vi "PrepForScan.vi"(0 "Motion Settings In":T1={"No Motion?"=FALSE, "Motion System"=enum."NI 735x", "Motion Bd ID"=1, "Motion Profile"="SMAC1", "# Axis"=1, "Reverse Z axis?"=TRUE, "SMAC Axis"=0, "scan pair"=enum."y-(x) scan", "RT fps"=6.0, "Steps per mm"=[1000, 1000, 1000, 1000], "Motor Parameters"={"velocity ct/s"=[10000.0, 10000.0, 10000.0, 50000.0], "accel ct/s^2"=[50000.0, 50000.0, 50000.0, 200000.0]}, "One Way Scan"=FALSE, "Reverse One Way Scan"=FALSE, "Global Position (mm)"=[], "Plane"=0, "Distance between\nscan lines (um)"=0.0, "Distance between\nscan planes (um)"=0.0, "number of scan planes"=1, "Total steps in line"=0, "Xtra plane\ndistance  (um)"=100, "Xtra planes "=1, "Add Axis"=FALSE, "overshoot cts"=200, "BKPT Shift"=0, "Scan Start Time (ms)"=0, "ESP VISA"="GPIB::1::INSTR", "3rd Axis"=1, "GL Ref Out"=refnum, "Galil Address"=""} {"3rd Axis" items=["x", "y", "z", "w"]; "Xtra planes" min=1; "Xtra plane\ndistance  (um)" min=0; "Distance between\nscan planes (um)" format="%.2f"; "Distance between\nscan lines (um)" format="%.2f"; "SMAC Axis" items=["None"=0, "Axis 1"=1, "Axis 2"=2, "Axis 3"=3, "Axis 4"=4, "Axis 5"=5, "Axis 6"=6, "Axis 7"=7, "Axis 8"=8, "Vector Space 1"=17, "Vector Space 2"=18, "Vector Space 3"=19, "Vector Space 4"=20]; "Motion Bd ID" min=1 max=32 step=1}, 1 "Pause?":bool, 7 "SMAC?":bool, 9 "Scan Axis":i8, 11 "MoveBack?":bool, 12 "Digitizer Settings":T5={"Digitizer delay (us) "=0.0, "rf points per line"=0, "lines per plane"=0, "Samp Rate (Hz)"=0.0, "Additional dig delay (us)"=0.0, "Voltage Scale"=0.0, "Pre-Looks"=0, "Offset delay (us)"=0.0, "bits A/D"=0, "Avg Num"=0, "DigTimeOut"=0.0, "Rel Dig Delay"=0.0, "Dig Ch"=0, "LeCroyCluster"={"LeCroy Channels"=[], "LC read pt offset"=0.0, "Sweep Avg"=FALSE}, "Main Digitizer"=enum."NI Digitizer", "Dig Config"=enum."Single channel", "Digitizer ID Cluster"={"Acqiris/Alazar/SP ID"=[], "NI Instr Handles"=[], "LeCroy VISA"="", "GaGe Handle"={"Handle"=0, "Sample size"=0, "Resolution"=0, "Offset"=0, "Channels"=0, "Boards"=0}, "ATS Ref"="ATS9350", "Acqiris Address"=["PCI::INSTR0"], "ADQRef"=refnum, "adq_cu_ptr"=refnum}, "Trigger Settings"={"Trig Source"=1, "Trig Coupling"=0, "Trig Slope"=0, "Level (mV)"=1500.0}, "Bulk Acq"=FALSE, "Bulk Start Indexes"=[], "Data Ref RF"=refnum, "NI ID/Channel"=[], "Total Dig CH"=1, "Xtra Ann Trig delay (us)"=10.0, "Fix Z Delay?"=FALSE, "One Way Transmission?"=FALSE, "Data Ref Log"=refnum} {"Trigger Settings"."Trig Slope" items=["Positive", "Negative"]; "Trigger Settings"."Level (mV)" format="%.2f"; "Trigger Settings"."Trig Coupling" items=["DC 1 MOhm", "AC 1 MOhm", "DC 50 Ohm", "AC 50 Ohm"]; "Trigger Settings"."Trig Source" items=["Chan 1", "External"]; "Rel Dig Delay" format="%.2f"; "DigTimeOut" format="%.2f"; "Avg Num" min=1; "Offset delay (us)" format="%.2f"; "Additional dig delay (us)" format="%.2f"; "Digitizer delay (us)" format="%.2f"}) -> (4 "Counts":dbl, 6 "Axis Resource out":u16(ring) items=["Axis Control"=0, "Axis 1"=1, "Axis 2"=2, "Axis 3"=3, "Axis 4"=4, "Axis 5"=5, "Axis 6"=6, "Axis 7"=7, "Axis 8"=8, "Vector Space Control"=16, "Vector Space 1"=17, "Vector Space 2"=18, "Vector Space 3"=19, "Vector Space 4"=20, "Encoder Control"=32, "Encoder 1"=33, "Encoder 2"=34, "Encoder 3"=35, "Encoder 4"=36, "Encoder 5"=37, "Encoder 6"=38, "Encoder 7"=39, "Encoder 8"=40, "DAC Channel 1"=49, "DAC Channel 2"=50, "DAC Channel 3"=51, "DAC Channel 4"=52, "DAC Channel 5"=53, "DAC Channel 6"=54, "DAC Channel 7"=55, "DAC Channel 8"=56, "Stepper Output 1"=65, "Stepper Output 2"=66, "Stepper Output 3"=67, "Stepper Output 4"=68, "Stepper Output 5"=69, "Stepper Output 6"=70, "Stepper Output 7"=71, "Stepper Output 8"=72, "ADC Channel 1"=81, "ADC Channel 2"=82, "ADC Channel 3"=83, "ADC Channel 4"=84, "ADC Channel 5"=85, "ADC Channel 6"=86, "ADC Channel 7"=87, "ADC Channel 8"=88], 8 "Bd ID Out":u8, 10 "Program ID":u8 format="%.0x", 14 "Axis Move Info":cluster{"Resource Output":u16, "Position":i32} {"Resource Output" items=["Axis Control"=0, "Axis 1"=1, "Axis 2"=2, "Axis 3"=3, "Axis 4"=4, "Axis 5"=5, "Axis 6"=6, "Axis 7"=7, "Axis 8"=8, "Vector Space Control"=16, "Vector Space 1"=17, "Vector Space 2"=18, "Vector Space 3"=19, "Vector Space 4"=20, "Encoder Control"=32, "Encoder 1"=33, "Encoder 2"=34, "Encoder 3"=35, "Encoder 4"=36, "Encoder 5"=37, "Encoder 6"=38, "Encoder 7"=39, "Encoder 8"=40, "DAC Channel 1"=49, "DAC Channel 2"=50, "DAC Channel 3"=51, "DAC Channel 4"=52, "DAC Channel 5"=53, "DAC Channel 6"=54, "DAC Channel 7"=55, "DAC Channel 8"=56, "Stepper Output 1"=65, "Stepper Output 2"=66, "Stepper Output 3"=67, "Stepper Output 4"=68, "Stepper Output 5"=69, "Stepper Output 6"=70, "Stepper Output 7"=71, "Stepper Output 8"=72, "ADC Channel 1"=81, "ADC Channel 2"=82, "ADC Channel 3"=83, "ADC Channel 4"=84, "ADC Channel 5"=85, "ADC Channel 6"=86, "ADC Channel 7"=87, "ADC Channel 8"=88]}, 15 "error out":errorcluster)   [LabVIEW 2022 SP3]
uses:
  Digitizers/-DigitizerRoutines/DigitizerSettings.ctl
  Digitizers/-DigitizerRoutines/Digitizer.ctl
  Digitizers/-DigitizerRoutines/DigConfig.ctl
  Digitizers/-DigitizerRoutines/DigitizerID.ctl
  C:/Windows/System32/ADQAPI_dotNet_helper.dll
  MotionParameters.ctl
  MotionSys.ctl
  -MotionRoutines/ScanAxis.ctl
  -MotionRoutines/3rdAxis.ctl
  Galil/Command Menu.ctl
  <instrlib>/Newport ESP301/Newport ESP301.lvlib
  <vilib>/Motion/FlexMotion/CustomControls/CustomControls.llb/Program.flx
  <vilib>/Motion/FlexMotion/CustomControls/CustomControls.llb/Axis To Control.flx
panel:
  # "1-D and 2-D B scan settings"
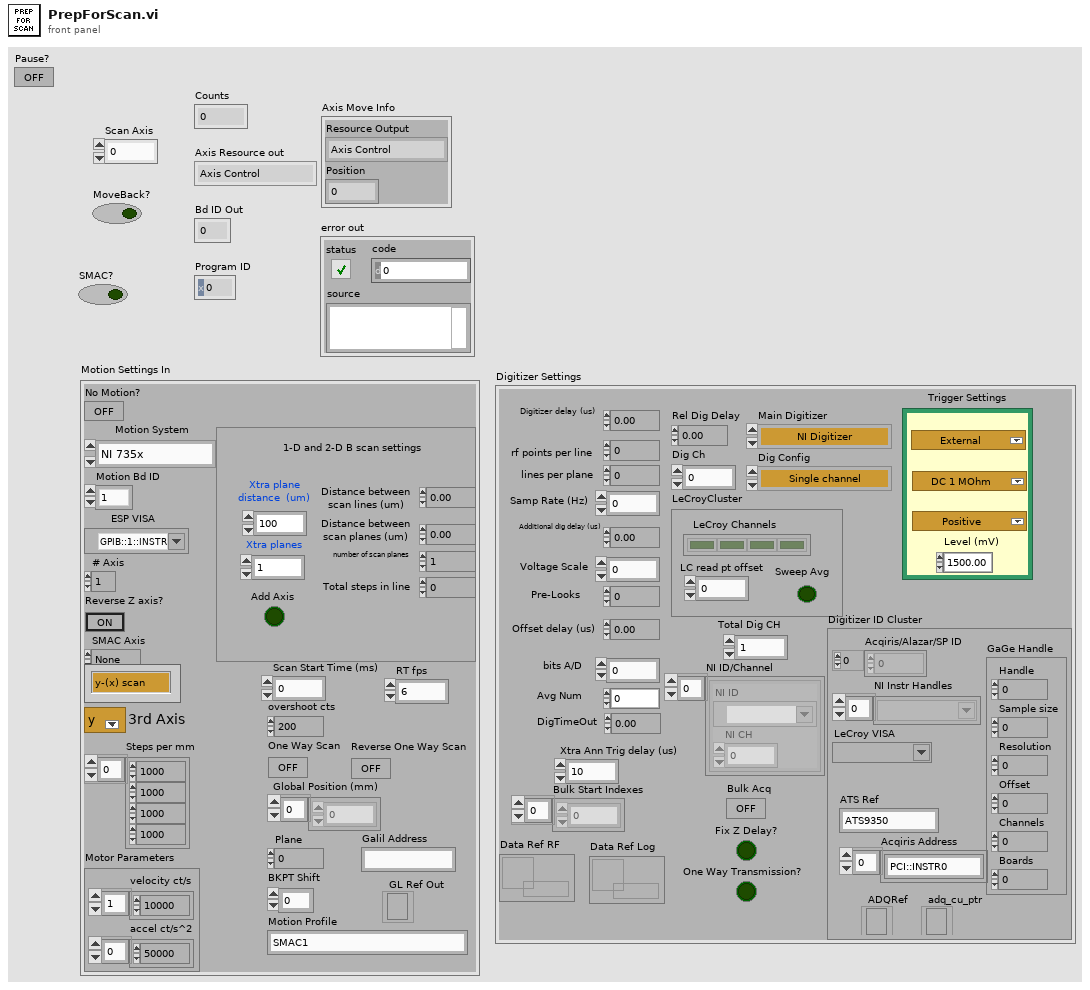
[diagram p1: front panel]
types:
  T1 = typedef "MotionParameters.ctl" = cluster{"No Motion?":bool, "Motion System":T2, "Motion Bd ID":u8, "Motion Profile":string, "# Axis":i8, "Reverse Z axis?":bool, "SMAC Axis":u16, "scan pair":T3, "RT fps":sgl, "Steps per mm":i32[], "Motor Parameters":cluster{"velocity ct/s":dbl[], "accel ct/s^2":dbl[]}, "One Way Scan":bool, "Reverse One Way Scan":bool, "Global Position (mm)":dbl[], "Plane":i32, "Distance between\nscan lines (um)":sgl, "Distance between\nscan planes (um)":sgl, "number of scan planes":i32, "Total steps in line":i32, "Xtra plane\ndistance  (um)":i32, "Xtra planes ":i32, "Add Axis":bool, "overshoot cts":i32, "BKPT Shift":i32, "Scan Start Time (ms)":u32, "ESP VISA":refnum<visa-resource-name>, "3rd Axis":T4, "GL Ref Out":refnum<k7>, "Galil Address":string}
  T2 = typedef "MotionSys.ctl" = enum16{"MM3000", "NI 735x", "Newport ESP", "No Motion Card", "Galil"}
  T3 = typedef "ScanAxis.ctl" = enum16{"y-(x) scan", "x-(y) scan", "z-(x) scan", "z-(y) scan", "y-(z) scan", "x-(z) scan", "w-(x) scan", "w-(y) scan", "w-(z) scan", "x-(w) scan", "y-(w) scan", "z-(w) scan"}
  T4 = typedef "3rdAxis.ctl" = u16
  T5 = typedef "DigitizerSettings.ctl" = cluster{"Digitizer delay (us) ":dbl, "rf points per line":i32, "lines per plane":i32, "Samp Rate (Hz)":dbl, "Additional dig delay (us)":dbl, "Voltage Scale":dbl, "Pre-Looks":i32, "Offset delay (us)":dbl, "bits A/D":i8, "Avg Num":i32, "DigTimeOut":sgl, "Rel Dig Delay":sgl, "Dig Ch":i32, "LeCroyCluster":cluster{"LeCroy Channels":bool[], "LC read pt offset":dbl, "Sweep Avg":bool}, "Main Digitizer":T6, "Dig Config":T7, "Digitizer ID Cluster":T8, "Trigger Settings":cluster{"Trig Source":u16, "Trig Coupling":u16, "Trig Slope":u16, "Level (mV)":dbl}, "Bulk Acq":bool, "Bulk Start Indexes":i32[], "Data Ref RF":refnum<data-value>, "NI ID/Channel":cluster{"NI ID":refnum<k15>, "NI CH":i32}[], "Total Dig CH":i32, "Xtra Ann Trig delay (us)":dbl, "Fix Z Delay?":bool, "One Way Transmission?":bool, "Data Ref Log":refnum<data-value>}
  T6 = typedef "Digitizer.ctl" = enum16{"Acqiris Digitizer", "NI Digitizer", "LeCroy", "GaGe", "AlazarTech", "No Digitizer", "Teledyne"}
  T7 = typedef "DigConfig.ctl" = enum16{"Single channel", "2 Chans w/ 2 Acqiris", "2 Chans w/ 1 Acqiris", "5-CH Pulser New", "5-CH pulser w/ ann array", "5-pass style ann array", "Empty"}
  T8 = typedef "DigitizerID.ctl" = cluster{"Acqiris/Alazar/SP ID":u32[], "NI Instr Handles":refnum<k15>[], "LeCroy VISA":refnum<visa-resource-name>, "GaGe Handle":cluster{"Handle":u32, "Sample size":u32, "Resolution":i32, "Offset":i32, "Channels":u32, "Boards":u32}, "ATS Ref":string, "Acqiris Address":string[], "ADQRef":refnum<k24>, "adq_cu_ptr":refnum<k24>}
  T9 = typedef "Resource Out (Enum).flx" = u16
  T10 = typedef "GL Axis Control.ctl" = u16
  T11 = typedef "Command Menu.ctl" = enum16{"CommandPassThrough", "Abort Motion", "Define Pos", "Velocity", "Acceleration", "Deceleration", "Position Rel", "Postion Abs", "Begin Move", "After Move", "Home", "KI", "KD", "KP", "IL", "Config I/O", "Set Bit", "Clear Bit", "Motor Off", "Moto On", "Status", "Execute", "Halt Execute", "HX Status", "Tell Velocity", "Check Motion", "BreakPoint", "Tell Position", "Current Code Line", "Tell Switches", "OC Force On", "OC Off", "Pos Soft Limit", "Rev Soft Limit"}
  T12 = typedef "Program.flx" = u8
  T13 = typedef "Bd Id Out" = u8
  T14 = typedef "Axis To Control.flx" = u16
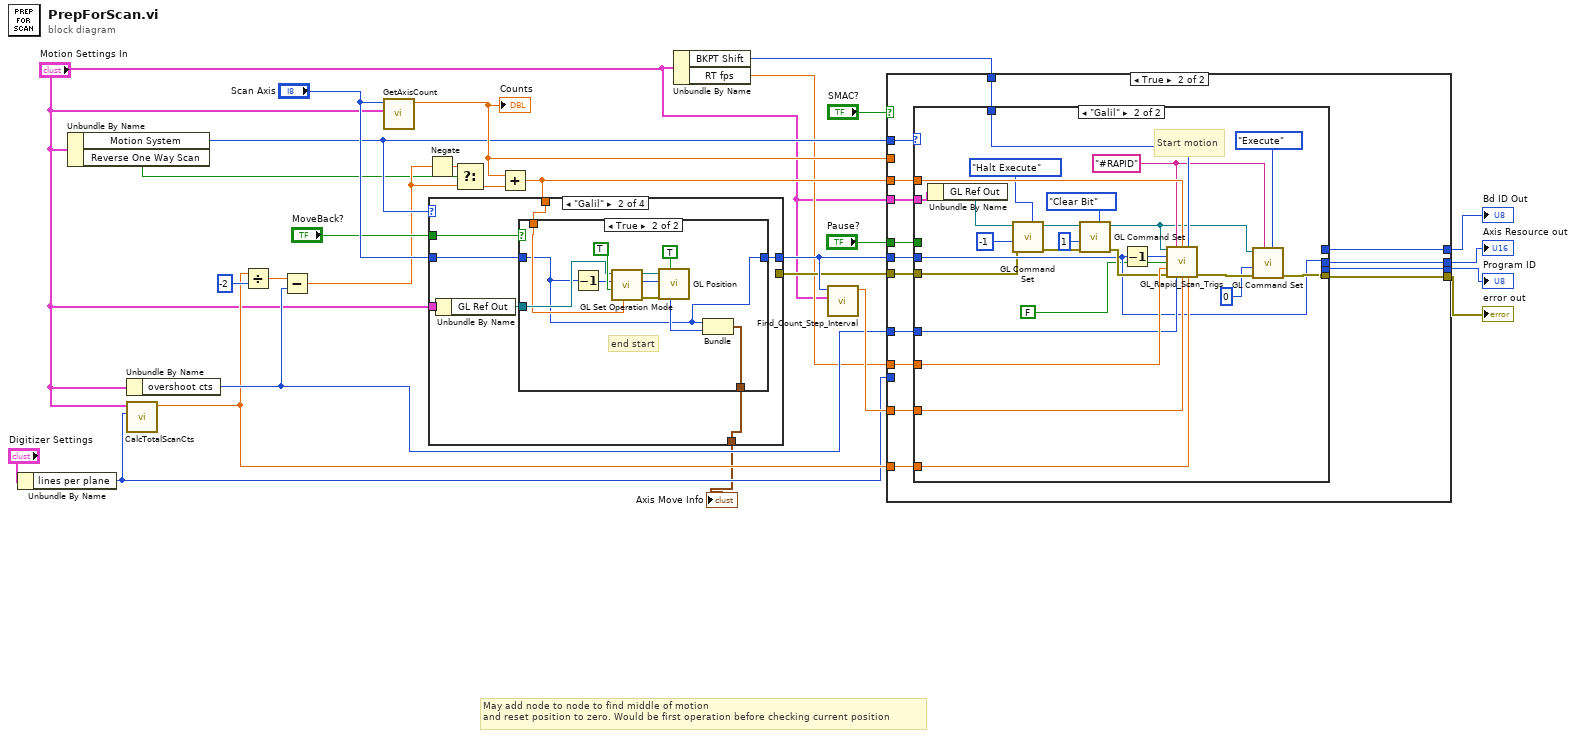
[diagram p0: block diagram]
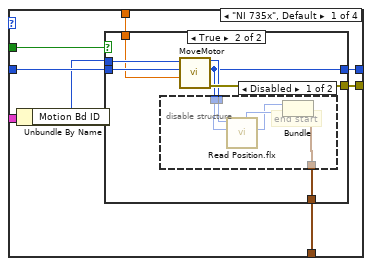
[diagram p2: hidden frame]
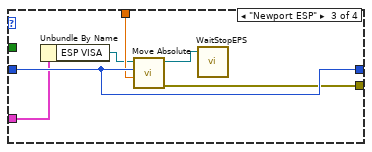
[diagram p6: hidden frame]
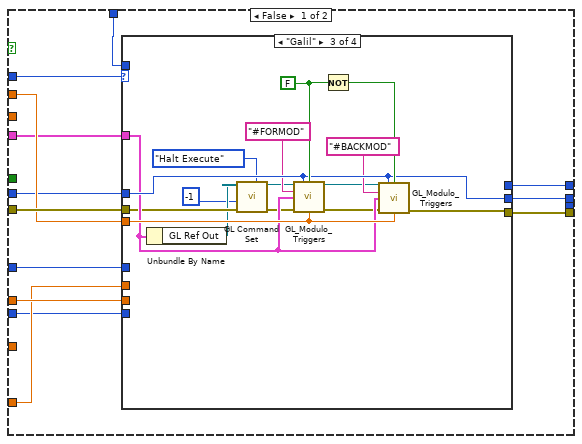
[diagram p8: hidden frame]
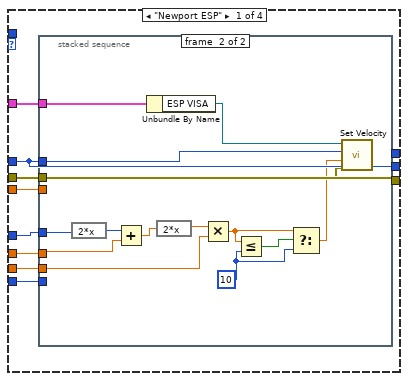
[diagram p9: hidden frame]
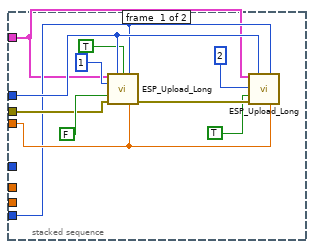
[diagram p10: hidden frame]
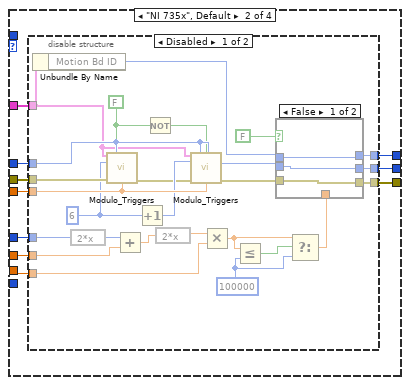
[diagram p11: hidden frame]
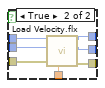
[diagram p12: hidden frame]
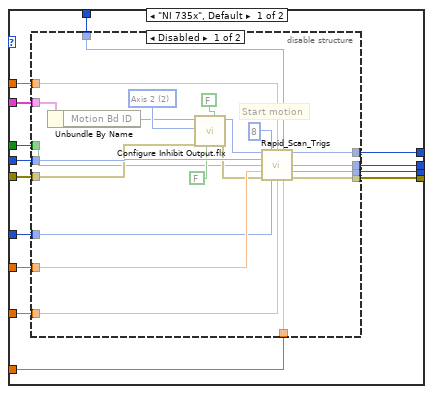
[diagram p15: hidden frame]
diagram:
  # "May add node to node to find middle of motion\nand reset position to zero. Would be first operation before checking current position"
  n1 = Unbundle By Name("Digitizer Settings") -> ("lines per plane"=w8:i32)
  n2 = Unbundle By Name("Motion Settings In") -> ("Motion System"=w13:T2, "Reverse One Way Scan"=w4:bool)
  n3 = Unbundle By Name("Motion Settings In") -> ("overshoot cts"=w12:i32)
  n4 = call "CalcTotalScanCts.vi"("Number of scan lines"=w8, "Motion Settings In"="Motion Settings In") -> ("Total Steps"=w9:dbl)  [unwired: 9 in]
  n5 = Divide(x=w9, y=-2) -> (x/y=w20:dbl)
  n6 = Subtract(x=w20, y=w12) -> (x-y=w6:dbl)
  n7 = call "GetAxisCount.vi"("Motion Settings"="Motion Settings In", "Scan Axis"="Scan Axis") -> ("Counts"=w28:dbl)  [unwired: 9 in]
  "Counts" <- w28
  n8 = Negate(x=w6) -> (-x=w5:dbl)
  n9 = Select(t=w5, s=w4, f=w6) -> (s? t:f=w7:dbl)
  n10 = Add(x=w28, y=w7) -> (x+y=w22:dbl)
  n11 = case shown="\"Galil\"" w13 {
    tunnel: [w35 w51 w74 _] -> w25
    tunnel: [w34 _ w72 _] -> w21
    tunnel: "Scan Axis" -> [w36 w56 w74 _]
    tunnel: w22 -> [w33 w55 w71 _]
    tunnel: "MoveBack?" -> [w32 w54 _ _]
    tunnel: "Motion Settings In" -> [w31 w53 w70 _]
    tunnel: [w29 w50 _ _] -> w2
    frame "NI 735x", Default {
      n12 = Unbundle By Name(w31) -> ("Motion Bd ID"=w30:u8)
      n13 = case shown="True" w32 {
        tunnel: w30 -> [_ w44]
        tunnel: w36 -> [w37 w43]
        tunnel: [w37 w39] -> w35
        tunnel: [_ w42] -> w34
        tunnel: w33 -> [_ w41]
        tunnel: [_ w38] -> w29
        frame False {
        }
        frame True {
          n14 = call "MoveMotor.vi"("Target Position (0)"=w41, "Axis or Vector Space"=w43, "Motion Bd ID"=w44) -> ("error out"=w42:errorcluster, "Resource Output"=w39:u16, "Bd ID Out"=w40:u8)  [unwired: 6 in]
          n15 = disable-structure shown="Disabled" {
            disable-tunnel: w40 -> [w47 _]
            disable-tunnel: w39 -> [w46 _]
            disable-tunnel: [w45 _] -> w38
            frame Disabled {
              # "end start"
              n16 = call <vilib>:"Read Position.flx"("Axis"=w46, "Board ID"=w47) -> ("Resource Output"=w48:T9, "Position"=w49:i32)  [unwired: 4 in, 2 out]
              n17 = Bundle("Resource Output"=w48, "Position"=w49) -> (w45:cluster{"Resource Output":T9, "Position":i32})  [unwired: 1 in]
            }
            frame Enabled {
            }
          }
        }
      }
    }
    frame "Galil" {
      n18 = Unbundle By Name(w53) -> ("GL Ref Out"=w52:refnum<k7>)
      n19 = case shown="True" w54 {
        tunnel: w56 -> [w57 w58]
        tunnel: w55 -> [_ w65]
        tunnel: w52 -> [_ w66]
        tunnel: [w57 w58] -> w51
        tunnel: [_ w59] -> w50
        frame False {
        }
        frame True {
          # "end start"
          n20 = Decrement(x=w58) -> (x-1=w61:i8)
          n21 = call "GL Set Operation Mode.vi"("position cts (abs/rel)"=w65, "Start Now?"=TRUE, "Axis"=w61, "Galil.IGalil"=w66) -> ("error out"=w63:errorcluster, "Axis Out Output"=w62:T10, "Galil Out"=w64:refnum<k7>)  [unwired: 5 in]
          n22 = call "GL Position.vi"("Wait for Motion Complete"=TRUE, "error in (no error)"=w63, "Axis"=w62, "Galil.IGalil"=w64) -> ("Axis Position"=w60:i32)  [unwired: 2 in, 3 out]
          n23 = Bundle("Scan Axis"=w58, "Axis Position"=w60) -> (w59:cluster{"Scan Axis":i8, "Axis Position":i32})  [unwired: 1 in]
        }
      }
    }
    frame "Newport ESP" {
      n24 = Unbundle By Name(w70) -> ("ESP VISA"=w69:refnum<visa-resource-name>)
      n25 = call <instrlib>:"Move Absolute.vi"("Position (0 units)"=w71, "Axis (1)"=w74, "VISA resource name"=w69) -> ("error out"=w72:errorcluster, "VISA resource name out"=w73:refnum<visa-resource-name>)  [unwired: 3 in]
      n26 = call "WaitStopEPS.vi"("VISA resource name"=w73) -> ()  [unwired: 2 in, 3 out]
    }
    frame "MM3000", "No Motion Card" {
    }
  }
  "Axis Move Info" <- w2
  n27 = Unbundle By Name("Motion Settings In") -> ("BKPT Shift"=w11:i32, "RT fps"=w10:sgl)
  n28 = call "Find_Count_Step_Interval.vi"("Motion Settings In"="Motion Settings In", "Axis"=w25) -> ("BP Interval"=w26:dbl)  [unwired: 8 in, 1 out]
  n29 = case shown="True" "SMAC?" {
    tunnel: w10 -> [w86 w198]
    tunnel: [w78 w197] -> w15
    tunnel: [w77 w196] -> w16
    tunnel: [_ w195] -> w18
    tunnel: [w75 w194] -> w19
    tunnel: w9 -> [w83 w193]
    tunnel: w26 -> [_ w192]
    tunnel: w12 -> [w87 w191]
    tunnel: w25 -> [w76 w190]
    tunnel: w21 -> [w85 w188]
    tunnel: w22 -> [_ w189]
    tunnel: w28 -> [w84 _]
    tunnel: w8 -> [w82 _]
    tunnel: w13 -> [w81 w185]
    tunnel: w11 -> [w80 w187]
    tunnel: "Motion Settings In" -> [w79 w186]
    tunnel: "Pause?" -> [_ w184]
    frame False {
      n30 = case shown="\"Galil\"" w81 {
        tunnel: w83 -> [w95 w130 _ _]
        tunnel: w76 -> [w90 w129 w178 w182]
        tunnel: w87 -> [w92 w128 _ _]
        tunnel: w86 -> [w91 w127 _ _]
        tunnel: w85 -> [w89 w126 w170 w183]
        tunnel: w84 -> [w93 w125 w181 _]
        tunnel: w82 -> [w94 _ _ _]
        tunnel: w80 -> [_ _ _ _]
        tunnel: w79 -> [w88 w121 w174 _]
        tunnel: [w89 w124 w172 w183] -> w78
        tunnel: [_ w123 _ _] -> w77
        tunnel: [w90 w122 w178 w182] -> w75
        frame "Newport ESP" {
          n31 = stacked-sequence {
            tunnel: w95 -> [_ w113]
            tunnel: w94 -> [w98 _]
            tunnel: w93 -> [w100 _]
            tunnel: w92 -> [_ w114]
            tunnel: w91 -> [_ w112]
            tunnel: w90 -> [w99 w110]
            tunnel: w89 -> [w103 w109]
            tunnel: w88 -> [w96 w108]
            frame #0 {
              n32 = call "ESP_Upload_Long.vi"("Motion Settings In"=w96, "Axis"=w99, "Purge?"=TRUE, "lines per scan"=w98, "Program#"=1, "Reverse ?"=FALSE, "error in"=w103, "Offset"=w100) -> ("error out"=w102:errorcluster)  [unwired: 6 in, 1 out]
              n33 = call "ESP_Upload_Long.vi"("Motion Settings In"=w96, "Axis"=w99, "lines per scan"=w98, "Program#"=2, "Reverse ?"=TRUE, "error in"=w102, "Offset"=w100) -> ()  [unwired: 7 in, 2 out]
            }
            frame #1 {
              w119 = 10
              n34 = expression code="2*x"(w114) -> (w117:i32)
              n35 = Add(x=w117, y=w113) -> (x+y=w115:dbl)
              n36 = Unbundle By Name(w108) -> ("ESP VISA"=w107:refnum<visa-resource-name>)
              n37 = expression code="2*x"(w115) -> (w116:dbl)
              n38 = Multiply(x=w116, y=w112) -> (x*y=w120:dbl)
              n39 = Less Or Equal?(x=w120, y=w119) -> (x <= y?=w118:bool)
              n40 = Select(t=w120, s=w118, f=w119) -> (s? t:f=w111:dbl)
              n41 = call <instrlib>:"Set Velocity.vi"("error in (no error)"=w109, "Velocity (units/s)"=w111, "Axis (1)"=w110, "VISA resource name"=w107) -> ()  [unwired: 2 in, 2 out]
            }
          }
        }
        frame "NI 735x", Default {
          n42 = disable-structure shown="Disabled" {
            disable-tunnel: w130 -> [w155 _]
            disable-tunnel: w129 -> [w154 _]
            disable-tunnel: w128 -> [w153 _]
            disable-tunnel: w127 -> [w152 _]
            disable-tunnel: w126 -> [w151 _]
            disable-tunnel: w125 -> [w150 _]
            disable-tunnel: [w149 _] -> w124
            disable-tunnel: [w134 _] -> w123
            disable-tunnel: [w133 _] -> w122
            disable-tunnel: w121 -> [w132 _]
            frame Disabled {
              w142 = 100000
              w145 = u8 6 ("Program (1)")
              w148 = FALSE
              n43 = Unbundle By Name(w132) -> ("Motion Bd ID"=w131:u8)
              n44 = expression code="2*x"(w153) -> (w140:i32)
              n45 = call "Modulo_Triggers.vi"("Motion Settings In"=w132, "Axis"=w154, "Reverse ?"=w148, "Program (1)"=w145, "error in (no error)"=w151, "Offset"=w150) -> ("error out"=w144:errorcluster)  [unwired: 3 in, 6 out]
              n46 = Add(x=w140, y=w155) -> (x+y=w138:dbl)
              n47 = Increment(x=w145) -> (x+1=w146:u8)
              n48 = Not(x=w148) -> (.not. x?=w147:bool)
              n49 = expression code="2*x"(w138) -> (w139:dbl)
              n50 = call "Modulo_Triggers.vi"("Motion Settings In"=w132, "Axis"=w154, "Reverse ?"=w147, "Program (1)"=w146, "error in (no error)"=w144, "Offset"=w150) -> ("error out"=w135:errorcluster)  [unwired: 3 in, 6 out]
              n51 = Multiply(x=w139, y=w152) -> (x*y=w143:dbl)
              n52 = Less Or Equal?(x=w143, y=w142) -> (x <= y?=w141:bool)
              n53 = Select(t=w143, s=w141, f=w142) -> (s? t:f=w137:dbl)
              n54 = case shown="False" FALSE {
                tunnel: w131 -> [w157 w165]
                tunnel: w154 -> [w156 w164]
                tunnel: w137 -> [_ w163]
                tunnel: [w158 w162] -> w149
                tunnel: w135 -> [w158 w161]
                tunnel: [w157 w160] -> w134
                tunnel: [w156 w159] -> w133
                frame False {
                }
                frame True {
                  n55 = call <vilib>:"Load Velocity.flx"("Velocity (10000)"=w163, "error in (no error)"=w161, "Axis or Vector Space"=w164, "Board ID"=w165) -> ("error out"=w162:errorcluster, "Resource Output"=w159:T9, "Bd ID Out"=w160:T13)  [unwired: 3 out]
                }
              }
            }
            frame Enabled {
            }
          }
        }
        frame "Galil" {
          w180 = FALSE
          n56 = Unbundle By Name(w174) -> ("GL Ref Out"=w168:refnum<k7>)
          n57 = call "GL Command Set.vi"("Command"=Command_Menu."Halt Execute", "error in (no error)"=w170, "Value"=-1, "Galil.IGalil"=w168) -> ("error out"=w171:errorcluster, "ref out"=w169:refnum<k7>)  [unwired: 3 in, 3 out]
          n58 = call "GL_Modulo_Triggers.vi"("GL Ref In"=w169, "Axis"=w178, "Reverse ?"=w180, "Program Name"="#FORMOD", "Motion Settings In"=w174, "error in"=w171, "Start Position"=w181) -> ("GL Ref Out"=w175:refnum<k7>, "error out"=w173:errorcluster)  [unwired: 6 in, 1 out]
          n59 = Not(x=w180) -> (.not. x?=w179:bool)
          n60 = call "GL_Modulo_Triggers.vi"("GL Ref In"=w175, "Axis"=w178, "Reverse ?"=w179, "Program Name"="#BACKMOD", "Motion Settings In"=w174, "error in"=w173, "Start Position"=w181) -> ("error out"=w172:errorcluster)  [unwired: 6 in, 2 out]
        }
        frame "MM3000", "No Motion Card" {
        }
      }
    }
    frame True {
      n61 = case shown="\"Galil\"" w185 {
        tunnel: w198 -> [w212 w258]
        tunnel: [w211 w246] -> w197
        tunnel: [w210 _] -> w196
        tunnel: [w209 _] -> w195
        tunnel: [w208 w242] -> w194
        tunnel: w193 -> [w207 w257]
        tunnel: w192 -> [w206 w256]
        tunnel: w191 -> [w205 w255]
        tunnel: w190 -> [w204 w242]
        tunnel: w189 -> [w203 w254]
        tunnel: w188 -> [w202 w238]
        tunnel: w187 -> [w201 w253]
        tunnel: w186 -> [w200 w252]
        tunnel: w184 -> [w199 _]
        frame "NI 735x", Default {
          n62 = disable-structure shown="Disabled" {
            disable-tunnel: w212 -> [w233 _]
            disable-tunnel: [w232 _] -> w211
            disable-tunnel: [w231 _] -> w210
            disable-tunnel: [w230 _] -> w209
            disable-tunnel: [w229 _] -> w208
            disable-tunnel: w207 -> [w228 _]
            disable-tunnel: w206 -> [w227 _]
            disable-tunnel: w205 -> [w226 _]
            disable-tunnel: w204 -> [w225 _]
            disable-tunnel: w203 -> [w224 _]
            disable-tunnel: w202 -> [w217 _]
            disable-tunnel: w201 -> [w216 _]
            disable-tunnel: w200 -> [w215 _]
            disable-tunnel: w199 -> [w213 _]
            frame Disabled {
              w219 = T14 2 items=["Axis 1"=1, "Axis 2"=2, "Axis 3"=3, "Axis 4"=4, "Axis 5"=5, "Axis 6"=6, "Axis 7"=7, "Axis 8"=8] ("Axis")
              # "Start motion"
              n63 = Unbundle By Name(w215) -> ("Motion Bd ID"=w214:u8)
              n64 = call <vilib>:"Configure Inhibit Output.flx"("Enable"=FALSE, "Polarity (Active Low)"=FALSE, "error in (no error)"=w217, "Axis"=w219, "Board ID"=w214) -> ("error out"=w222:errorcluster, "Bd ID Out"=w223:T13)  [unwired: 1 in, 4 out]
              n65 = call "Rapid_Scan_Trigs.vi"("Board ID"=w223, "Program (1)"=T12 8, "Start Position"=w224, "BKPT Shift"=w216, "Scan Axis"=w225, "Pause?"=w213, "# frames/ s"=w233, "error in (no error)"=w222, "overshoot"=w226, "step interval"=w227, "Total Steps (one way)"=w228) -> ("Bd ID Out"=w231:u8, "Axis Resource out"=w229:u16, "Program ID"=w230:u8, "error out"=w232:errorcluster)  [unwired: 1 out]
            }
            frame Enabled {
            }
          }
        }
        frame "Galil" {
          w245 = "#RAPID" ("Program Name")
          # "Start motion"
          n66 = Unbundle By Name(w252) -> ("GL Ref Out"=w236:refnum<k7>)
          n67 = call "GL Command Set.vi"("Command"=Command_Menu."Halt Execute", "error in (no error)"=w238, "Value"=-1, "Galil.IGalil"=w236) -> ("error out"=w239:errorcluster, "ref out"=w237:refnum<k7>)  [unwired: 3 in, 3 out]
          n68 = call "GL Command Set.vi"("Command"=Command_Menu."Clear Bit", "error in (no error)"=w239, "Value"=1, "Galil.IGalil"=w237) -> ("error out"=w249:errorcluster, "ref out"=w244:refnum<k7>)  [unwired: 3 in, 3 out]
          n69 = Decrement(x=w242) -> (x-1=w243:u16)
          n70 = call "GL_Rapid_Scan_Trigs.vi"("GL Ref Out"=w244, "Program Name"=w245, "Start Position"=w254, "BKPT Shift"=w253, "Axis"=w243, "Pause?"=FALSE, "# frames/ s"=w258, "error in"=w249, "overshoot"=w255, "step interval"=w256, "Total Steps (one way)"=w257) -> ("error out"=w247:errorcluster)  [unwired: 2 in, 2 out]
          n71 = call "GL Command Set.vi"("Command"=Command_Menu."Execute", "Text Input"=w245, "error in (no error)"=w247, "Value"=0, "Galil.IGalil"=w244) -> ("error out"=w246:errorcluster)  [unwired: 2 in, 4 out]
        }
      }
    }
  }
  "Axis Resource out" <- w19
  "Program ID" <- w18
  "Bd ID Out" <- w16
  "error out" <- w15
